vi "ArdnoGetValveNums.vi"() -> (3 "Array":i32[](array[numeric]))   [LabVIEW 2018, in "Arduino.lvlib"]
uses:
  Arduino.lvlib
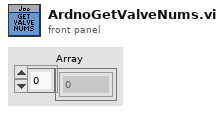
[diagram p1: front panel]
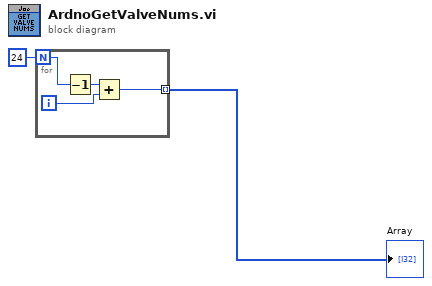
[diagram p0: block diagram]
diagram:
  n1 = for {
    N: 24 -> [w6]
    tunnel: [w3] -> w2 mode=indexing
    i -> [w4]
    n2 = Decrement(x=w6) -> (x-1=w5:i32)
    n3 = Add(x=w5, y=w4) -> (x+y=w3:i32)
  }
  "Array" <- w2
